vi "programmatic cluster value test.vi"() -> ()   [LabVIEW 2013]
panel:
  out "Array 2":u32[](array[numeric])
  out "Array":string[](array[string])
  out "String":string
  in  "Search Val":string
  in  "Cluster":T1 {"Slide" scale=0.0..10.0}
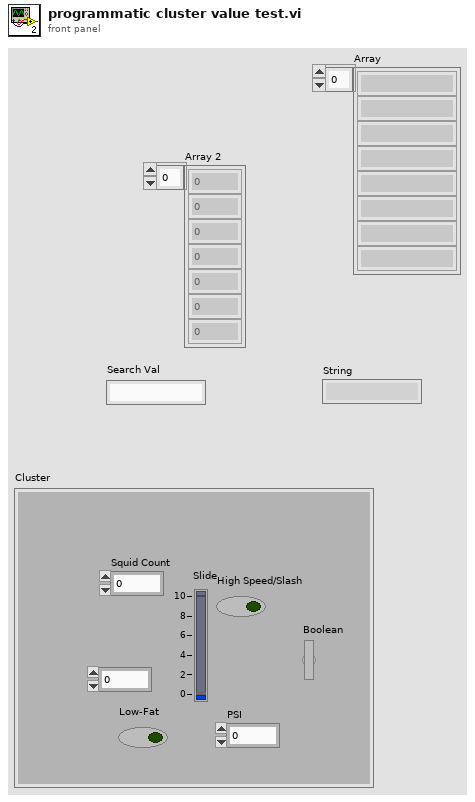
[diagram p1: front panel]
types:
  T1 = cluster{"PSI":dbl, "Low-Fat":bool, "Squid Count":ext, "High Speed/Slash":bool, dbl, "Boolean":bool, "Slide":dbl}
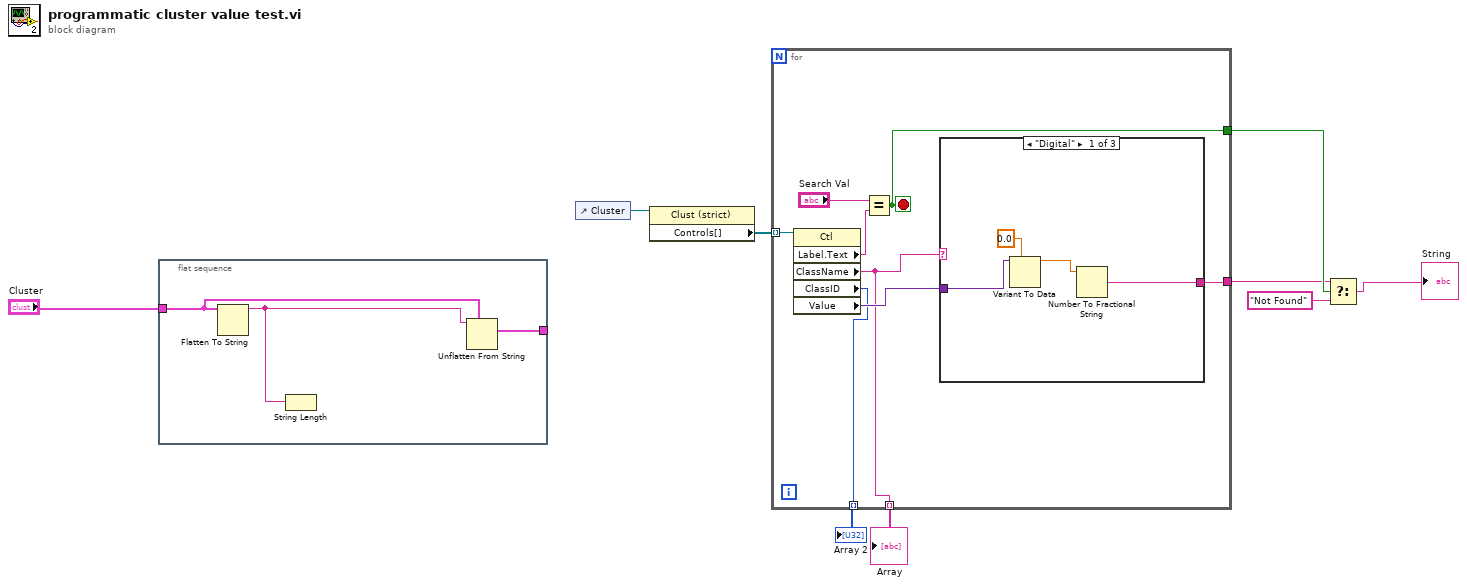
[diagram p0: block diagram]
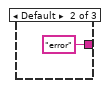
[diagram p2: hidden frame]
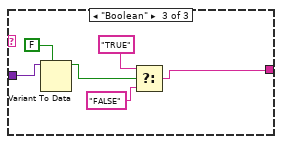
[diagram p3: hidden frame]
diagram:
  n1 = flat-sequence {
    tunnel: [w11] -> _
    tunnel: "Cluster" -> [w10]
    frame #0 {
      n2 = Flatten To String(anything=w10) -> (data string=w12:string)  [unwired: 3 in, 2 out]
      n3 = String Length(string=w12) -> ()  [unwired: 1 out]
      n4 = Unflatten From String(type=w10, binary string=w12) -> (value=w11:T1)  [unwired: 3 in, 2 out]
    }
  }
  n5 = control-ref of="Cluster"() -> (w8:refnum<vi>)
  n6 = property class="Clust (strict)"(reference=w8) -> ("Controls[]"=w7:refnum<vi>[])  [unwired: 1 in, 2 out]
  n7 = for {
    tunnel: w7 -> [w20] mode=indexing
    tunnel: [w17] -> w4
    tunnel: [w14] -> w6 mode=indexing
    tunnel: [w15] -> w5
    tunnel: [w13] -> w1 mode=indexing
    stop <- w15 stop-if-true
    n8 = property class="Ctl"(reference=w20) -> ("Label.Text"=w16:string, "ClassName"=w14:string, "ClassID"=w13:u32, "Value"=w18:variant)  [unwired: 1 in, 2 out]
    n9 = Equal?(x="Search Val", y=w16) -> (x = y?=w15:bool)
    n10 = case shown="\"Digital\"" w14 {
      tunnel: w18 -> [w24 _ w31]
      tunnel: [w21 "error" w26] -> w17
      frame "Digital" {
        n11 = Variant To Data(type=0.0, Variant=w24) -> (data=w22:dbl)  [unwired: 1 in, 1 out]
        n12 = Number To Fractional String(number=w22) -> (F-format string=w21:string)  [unwired: 3 in]
      }
      frame Default {
      }
      frame "Boolean" {
        n13 = Variant To Data(type=FALSE, Variant=w31) -> (data=w29:bool)  [unwired: 1 in, 1 out]
        n14 = Select(t="TRUE", s=w29, f="FALSE") -> (s? t:f=w26:string)
      }
    }
  }
  "Array" <- w6
  "Array 2" <- w1
  n15 = Select(t=w4, s=w5, f="Not Found") -> (s? t:f=→"String":string)
